vi "Configure Data.vi"(7 "DataArray":dbl[](array[numeric])=[0.0] format="%.2p", 8 "error in (no error)":errorcluster {"code" format="%.0x"}, 10 "RepCapIdentifier":string="Antenna" caption="RepCapIdentifier (Antenna)", 11 "instrument handle":refnum<k15>) -> (0 "error out":errorcluster {"code" format="%.0x"}, 3 "instrument handle out":refnum<k15>)   [LabVIEW 2009, in "Keysight XSAn.lvlib"]
doc: "Replaces and Configures all existing the correction points in the specified set.\n\nSupported Models: All supported"
uses:
  <instrlib>/Keysight XSAn/Keysight XSAn.lvlib
  AgXSAn.dll
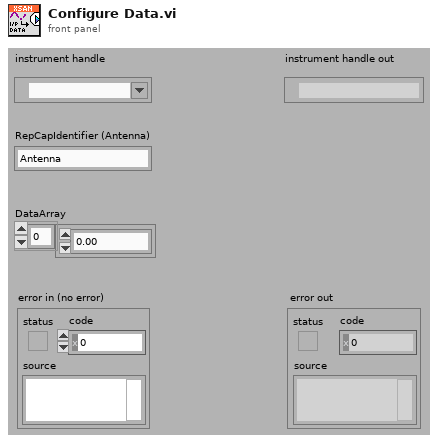
[diagram p1: front panel]
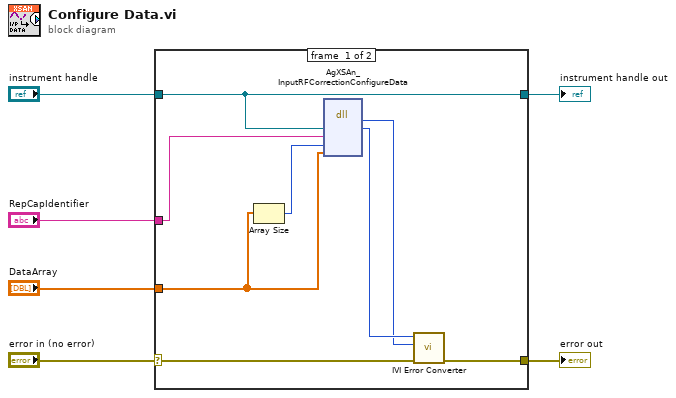
[diagram p0: block diagram]
diagram:
  n1 = case shown="No Error" "error in (no error)" {
    selector: "error in (no error)" -> [w12 w16]
    tunnel: [w11 w16] -> w6
    tunnel: "instrument handle" -> [w9 w15]
    tunnel: "RepCapIdentifier" -> [w10 _]
    tunnel: "DataArray" -> [w7 _]
    tunnel: [w9 w15] -> w1
    frame #0 {
      n2 = Array Size(array=w7) -> (size(s)=w8:i32)
      n3 = dll-call lib="AgXSAn**.dll" fn="AgXSAn_InputRFCorrectionConfigureData"("Vi"=w9, "RepCapIdentifier"=w10, "DataArrayBufferSize"=w8, "DataArray"=w7) -> (w13:i32, "Vi"=w14:u32)  [unwired: 6 in, 2 out]
      n4 = call <instrlib>:"IVI Error Converter.vi"("error in (no error)"=w12, "IVI error code (0)"=w13, "instrument handle"=w14) -> ("error out"=w11:errorcluster)  [unwired: 7 in, 1 out]
    }
    frame #1 {
    }
  }
  "error out" <- w6
  "instrument handle out" <- w1
